vi "detrend_line.vi"(11 "data_in":dbl[](array[numeric])) -> (3 "detrended":dbl[](array[numeric]))   [LabVIEW 2017]
uses:
  <vilib>/Analysis/NI_AALPro.lvlib
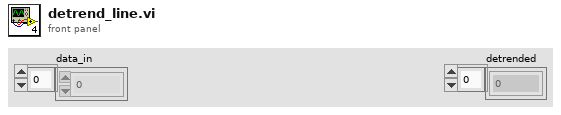
[diagram p1: front panel]
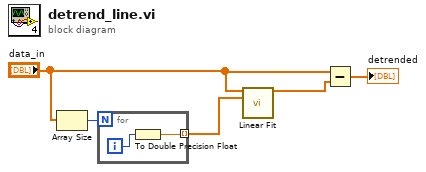
[diagram p0: block diagram]
diagram:
  n1 = Array Size(array="data_in") -> (size(s)=w5:i32)
  n2 = for {
    N: w5 -> [_]
    tunnel: [w6] -> w4 mode=indexing
    i -> [w7]
    n3 = To Double Precision Float(number=w7) -> (double precision float=w6:dbl)
  }
  n4 = call <vilib>:"Linear Fit.vi"("Y"="data_in", "X"=w4) -> ("Best Linear Fit"=w2:dbl[])  [unwired: 9 in, 4 out]
  n5 = Subtract(x="data_in", y=w2) -> (x-y=→"detrended":dbl[])
